vi "AlazarConfigureSampleSkipping.vi"(0 "Handle":u64, 5 "Mode":u32(ring) items=["Disable", "Enable"], 7 "Sample Clocks Per Record":u32, 9 "Sample Skip Bitmap":u16[](array[numeric]), 11 "error in (no error)":errorcluster) -> (4 "Handle":u64, 10 "Return Code":u32, 15 "error out":errorcluster)   [LabVIEW 2018]
doc: "Use this function to allow the digitizer to sub-sample post trigger data in arbitrary, non-uniform intervals. The application specifies which sample clock edges after a trigger event that the digitizer should use to generate sample points, and which sample clock edges that the digitizer should ignore."
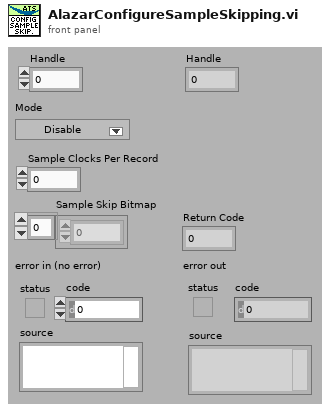
[diagram p1: front panel]
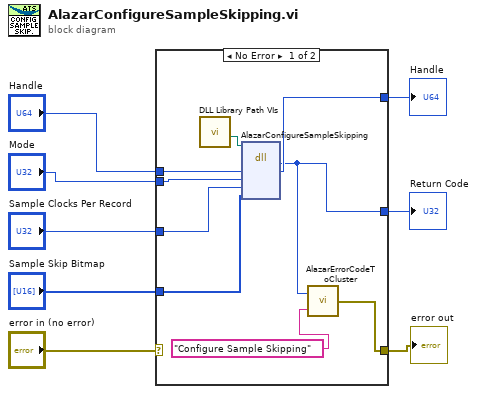
[diagram p0: block diagram]
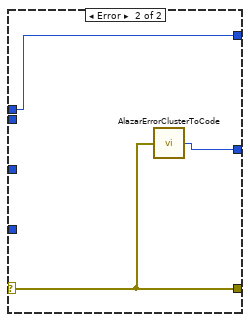
[diagram p2: hidden frame]
diagram:
  n1 = case shown="No Error" "error in (no error)" {
    selector: "error in (no error)" -> [_ w20]
    tunnel: [w11 w20] -> w7
    tunnel: "Handle" -> [w17 w19]
    tunnel: [w16 w19] -> w5
    tunnel: "Mode" -> [w15 _]
    tunnel: "Sample Clocks Per Record" -> [w14 _]
    tunnel: "Sample Skip Bitmap" -> [w13 _]
    tunnel: [w12 w18] -> w1
    frame No Error {
      n2 = call "DLL Library Path VIs.vi"() -> ("Alazar"=w9:path)  [unwired: 9 in, 2 out]
      n3 = dll-call lib="C:/Project/SerialSectOCT - FFT GPU/SerialSectOCT/Labview Software/DLL/ATSApi.dll" fn="AlazarConfigureSampleSkipping"(path in=w9, "handle"=w17, "Mode"=w15, "sampleClocksPerSecond"=w14, "pSampleSkipBitmap"=w13) -> ("return type"=w12:u32, "handle"=w16:u64)  [unwired: 5 in, 2 out]
      n4 = call "AlazarErrorCodeToCluster.vi"("Message"="Configure Sample Skipping", "Error Code"=w12) -> ("error out"=w11:errorcluster)
    }
    frame Error {
      n5 = call "AlazarErrorClusterToCode.vi"("error in (no error)"=w20) -> ("Error Code"=w18:u32)
    }
  }
  "Handle" <- w5
  "error out" <- w7
  "Return Code" <- w1
